vi "WPI_DualCameraBackground Loop.vi"(10 "BackCameraDevRef":T1, 11 "FrontCameraDevRef":T1) -> ()   [LabVIEW 2016]
doc: "This VI acquires the image buffer from the camera MJPG stream at the configured fps rate. It notifies any waiting VIs and allows them to pick up the latest image. This allows the camera and robot vision loop to run at different rates. The 1011, camera is far more efficient using MJPGs, and generally, this is probably the better choice for the camera loop.\n \nThis software is licensed. Open the labview\\readme\\WPI Robotics Library Open Source License.txt file for more information."
uses:
  <vilib>/Rock Robotics/WPI/Camera/WPI_CameraDevRef.ctl
  <vilib>/Rock Robotics/WPI/Camera/WPI_CameraSettings Operations.ctl
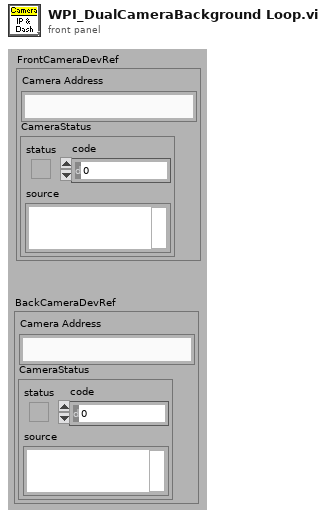
[diagram p1: front panel]
types:
  T1 = typedef "WPI_CameraDevRef.ctl" = cluster{"Camera Address":string, "CameraStatus":errorcluster}
  T2 = typedef "WPI_CameraSettings Operations.ctl" = enum16{"Udate FPS", "Update Compression", "Update Size", "Update White Balance", "Update Brightness", "Update Sharpness", "Update Exposure", "Update Exposure Value", "Update Color Level", "Update Exp Priority", "Update Color Enable", "Update JPG", "Update MJPG", "Read and Clear", "Read", "Init"}
  T3 = typedef "WPI_CameraSettings Control.ctl" = cluster{"FPS":i32, "Compression":i32, "Size":i32, "White Balance":i32, "Brightness":i32, "Sharpness":i32, "Exposure":i32, "Color Level":i32, "Exposure Priority":i32, "Color Enable":i32, "JPG Loop":i32, "MJPG Loop":i32, "Exposure Value":i32}
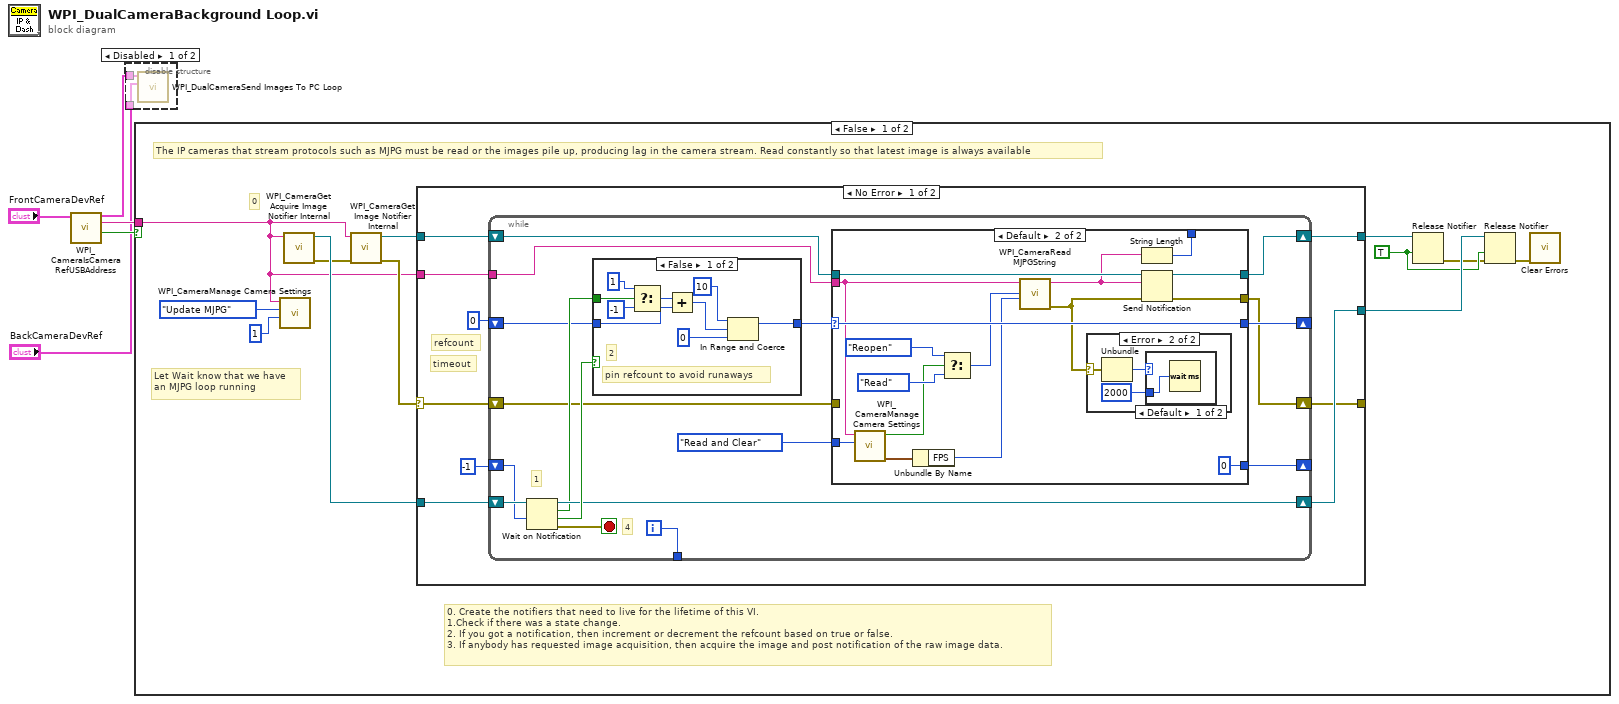
[diagram p0: block diagram]
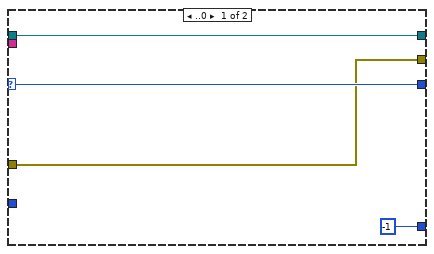
[diagram p3: hidden frame]
diagram:
  n1 = call <vilib>:"WPI_CameraIsCameraRefUSBAddress.vi"("CameraDevRef"="FrontCameraDevRef") -> ("USB?"=w4:bool, "Camera Address Out"=w3:string, "CameraDevRef out"=w2:T1)  [unwired: 7 in, 1 out]
  n2 = disable-structure shown="Disabled" {
    disable-tunnel: w2 -> [w7 _]
    disable-tunnel: "BackCameraDevRef" -> [w6 _]
    frame Disabled {
      n3 = call "WPI_DualCameraSend Images To PC Loop.vi"("BackCameraDevRef"=w6, "FrontCameraDevRef"=w7) -> ()  [unwired: 10 in]
    }
    frame Enabled {
    }
  }
  n4 = case shown="False" w4 {
    tunnel: w3 -> [w9 _]
    frame False {
      w16 = TRUE ("force destroy? (F)")
      # "The IP cameras that stream protocols such as MJPG must be read or the images pile up, producing lag in the camera stream. Read constantly so that latest image is always available"
      # "0. Create the notifiers that need to live for the lifetime of this VI. \n1.Check if there was a state change.\n2. If you got a notification, then increment or decrement the refcount based on true or false.\n3. If anybody has requested image acquisition, then acquire the image and post notification of the raw image data."
      # "Let Wait know that we have\nan MJPG loop running"
      # "0"
      n5 = call <vilib>:"WPI_CameraManage Camera Settings.vi"("Value"=1, "Operation"=WPI_CameraSettings_Operations."Update MJPG", "Camera IP"=w9) -> ()  [unwired: 7 in, 2 out]
      n6 = call <vilib>:"WPI_CameraGet Acquire Image Notifier Internal.vi"("Camera Address"=w9) -> ("error out"=w13:errorcluster, "Acquire Image Notifier"=w14:refnum<notifier>)  [unwired: 1 in, 8 out]
      n7 = call <vilib>:"WPI_CameraGet Image Notifier Internal.vi"("error in (no error)"=w13, "Camera Address"=w9) -> ("error out"=w15:errorcluster, "Image Notifier"=w17:refnum<notifier>)  [unwired: 8 out]
      n8 = case shown="No Error" w15 {
        selector: w15 -> [w21 w82]
        tunnel: w9 -> [w28 _]
        tunnel: w14 -> [w27 w80]
        tunnel: w17 -> [w25 w81]
        tunnel: [w23 w81] -> w19
        tunnel: [w22 w80] -> w18
        tunnel: [w20 w82] -> _
        frame No Error {
          # "timeout"
          # "refcount"
          n9 = while {
            shift-right: [w43] -> w22
            shift-left: w27 -> [w45]
            tunnel: w28 -> [w40]
            shift-right: [w32] -> _
            shift-left: 0 -> [w41]
            shift-right: [w38] -> w23
            shift-left: w25 -> [w39]
            shift-right: [w36] -> _
            shift-left: -1 -> [w37]
            shift-right: [w31] -> w20
            shift-left: w21 -> [w34]
            tunnel: [w29] -> _
            i -> [w29]
            stop <- w35 stop-if-true
            # "4"
            # "1"
            n10 = Wait on Notification(notifier=w45, timeout in ms (-1)=w37) -> (notifier out=w43:refnum<notifier>, notification=w42:bool, timed out?=w44:bool, error out=w35:errorcluster)  [unwired: 1 in, 1 out]
            n11 = case shown="False" w44 {
              tunnel: w42 -> [w78 _]
              tunnel: w41 -> [w74 w79]
              tunnel: [w70 w79] -> w33
              frame False {
                # "pin refcount to avoid runaways"
                # "2"
                n12 = Select(t=1, s=w78, f=-1) -> (s? t:f=w75:i32)
                n13 = Add(x=w75, y=w74) -> (x+y=w71:i32)
                n14 = In Range and Coerce(upper limit=10, x=w71, lower limit=0) -> (coerced(x)=w70:i32)  [unwired: 1 out]
              }
              frame True {
              }
            }
            n15 = case shown="Default" w33 {
              selector: w33 -> [w48 w62]
              tunnel: w40 -> [_ w50]
              tunnel: w39 -> [w49 w65]
              tunnel: [w49 w64] -> w38
              tunnel: [-1 0] -> w36
              tunnel: w34 -> [w46 _]
              tunnel: [w48 w62] -> w32
              tunnel: [w46 w61] -> w31
              tunnel: [_ w55] -> _
              tunnel: WPI_CameraSettings_Operations."Read and Clear" ("Operation") -> [_ w51]
              frame ..0 {
              }
              frame Default {
                n16 = call <vilib>:"WPI_CameraManage Camera Settings.vi"("Operation"=w51, "Camera IP"=w50) -> ("Values"=w53:T3, "Changed"=w54:bool)  [unwired: 8 in]
                n17 = Unbundle By Name(w53) -> ("FPS"=w52:i32)
                n18 = Select(t=enum16{"Read", "Reopen", "Close"}."Reopen" ("Operation"), s=w54, f=enum16{"Read", "Reopen", "Close"}."Read" ("Operation")) -> (s? t:f=w57:enum16{"Read", "Reopen", "Close"})
                n19 = call <vilib>:"WPI_CameraRead MJPGString.vi"("fps"=w52, "Operation"=w57, "address"=w50) -> ("error out"=w60:errorcluster, "Raw Image Data"=w56:string)  [unwired: 7 in]
                n20 = case shown="Error" w60 {
                  selector: w60 -> [_ w68]
                  frame No Error {
                  }
                  frame Error {
                    n21 = Unbundle(w68) -> ("code"=w67:i32)  [unwired: 2 out]
                    n22 = case shown="Default" w67 {
                      tunnel: u32 2000 ("milliseconds to wait") -> [w69 _]
                      frame Default {
                        n23 = Wait (ms)(milliseconds to wait=w69) -> ()  [unwired: 1 out]
                      }
                      frame 56 {
                      }
                    }
                  }
                }
                n24 = String Length(string=w56) -> (length=w55:i32)
                n25 = Send Notification(notification=w56, notifier=w65, error in (no error)=w60) -> (notifier out=w64:refnum<notifier>, error out=w61:errorcluster)
              }
            }
          }
        }
        frame Error {
        }
      }
      n26 = Release Notifier(notifier=w19, force destroy? (F)=w16) -> (error out=w12:errorcluster)  [unwired: 1 in, 2 out]
      n27 = Release Notifier(notifier=w18, force destroy? (F)=w16, error in (no error)=w12) -> (error out=w8:errorcluster)  [unwired: 2 out]
      n28 = call <vilib>:"Clear Errors.vi"("error in (no error)"=w8) -> ()  [unwired: 1 in, 6 out]
    }
    frame True {
      # "The USB cameras may need to be forwarded over ethernet. Read, compress, and send to the Dashbd."
    }
  }
